vi "Keithley 2400 Read.vi"(7 "Read Type":enum16{"Voltage", "Current"}(ring), 8 "error in (no error)":errorcluster, 11 "VISA Refnum in":refnum<visa-resource-name>) -> (0 "error out":errorcluster, 3 "Voltage Reading":dbl)   [LabVIEW 2019]
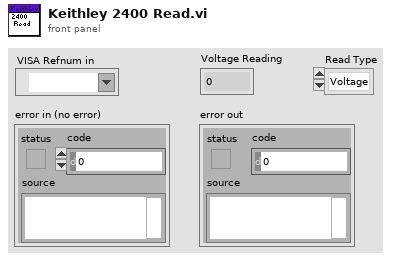
[diagram p1: front panel]
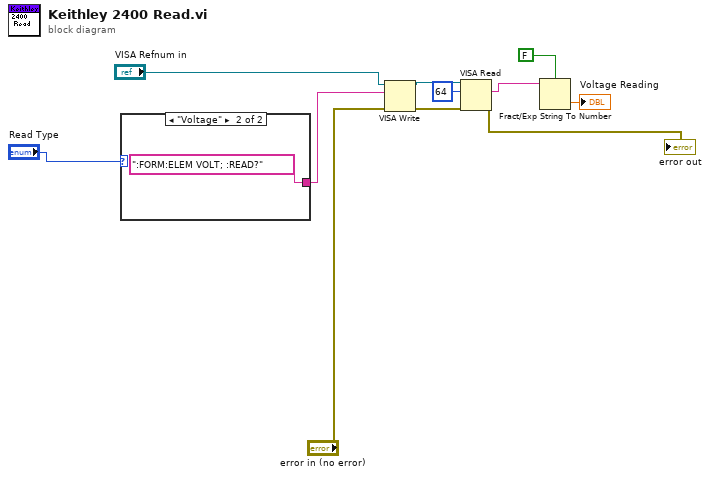
[diagram p0: block diagram]
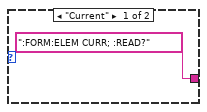
[diagram p2: hidden frame]
diagram:
  n1 = case shown="\"Voltage\"" "Read Type" {
    tunnel: [":FORM:ELEM CURR; :READ?" ("write buffer") ":FORM:ELEM VOLT; :READ?" ("write buffer")] -> w1
    frame "Current" {
    }
    frame "Voltage" {
    }
  }
  n2 = VISA Write(VISA resource name="VISA Refnum in", write buffer=w1, error in (no error)="error in (no error)") -> (VISA resource name out=w7:refnum<visa-resource-name>, error out=w6:errorcluster)  [unwired: 1 out]
  n3 = VISA Read(VISA resource name=w7, byte count=u32 64, error in (no error)=w6) -> (read buffer=w9:string, error out=→"error out":errorcluster)  [unwired: 2 out]
  n4 = Fract/Exp String To Number(use system decimal point (T)=FALSE, string=w9) -> (number=→"Voltage Reading":dbl)  [unwired: 2 in, 1 out]
